vi "Copy Test.vi"(4 "New ID":string, 6 "Move?":bool, 7 "New Parent ID":string, 8 "error in (no error)":errorcluster, 9 "Insertion Index":i32=-1, 10 "Test ID":string, 11 "Test Executive in":refnum<class "Test Executive.lvclass">) -> (0 "error out":errorcluster, 2 "Test ID out":string, 3 "Test Executive out":refnum<class "Test Executive.lvclass">)   [LabVIEW 2019, in "Test Executive.lvlib" / "Test Executive.lvclass"]
uses:
  <vilib>/gpm_packages/@cs/test-executive/Source/Test Executive/TestExecutive/Test Executive.lvclass
  <vilib>/gpm_packages/@cs/test-executive/Source/Test Executive/Executioner/Executioner.lvclass
  <vilib>/gpm_packages/@cs/test-executive/Source/Test Executive/TestExecutive/Test Executive.lvclass/Test Executive.ctl
  a368e383-e4da-4751-aab3-72c07474878c.vi
  fd6f22e2-1d92-4eb3-b93e-b19a74c7291f.vi
  b72c362c-b0aa-47de-9306-dfc13f43c4ad.vi
  cb6e558c-ce6a-4807-984b-722166e3a381.vi
  3584d46b-2973-4467-aaf0-07419839f110.vi
  <vilib>/gpm_packages/@cs/linked-list/Source/Linked List/ILinkedList/ILinked List.lvclass
  <vilib>/gpm_packages/@cs/linked-list/Source/Linked List/Linked List Ref/Linked List Ref.lvclass
panel:
  out "Data IDs out":variant
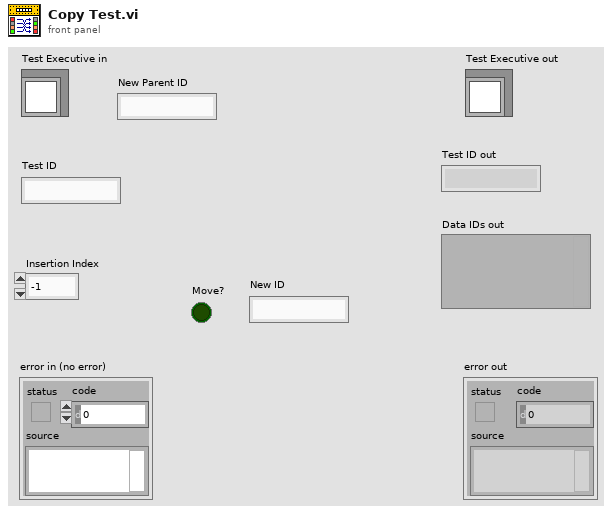
[diagram p1: front panel]
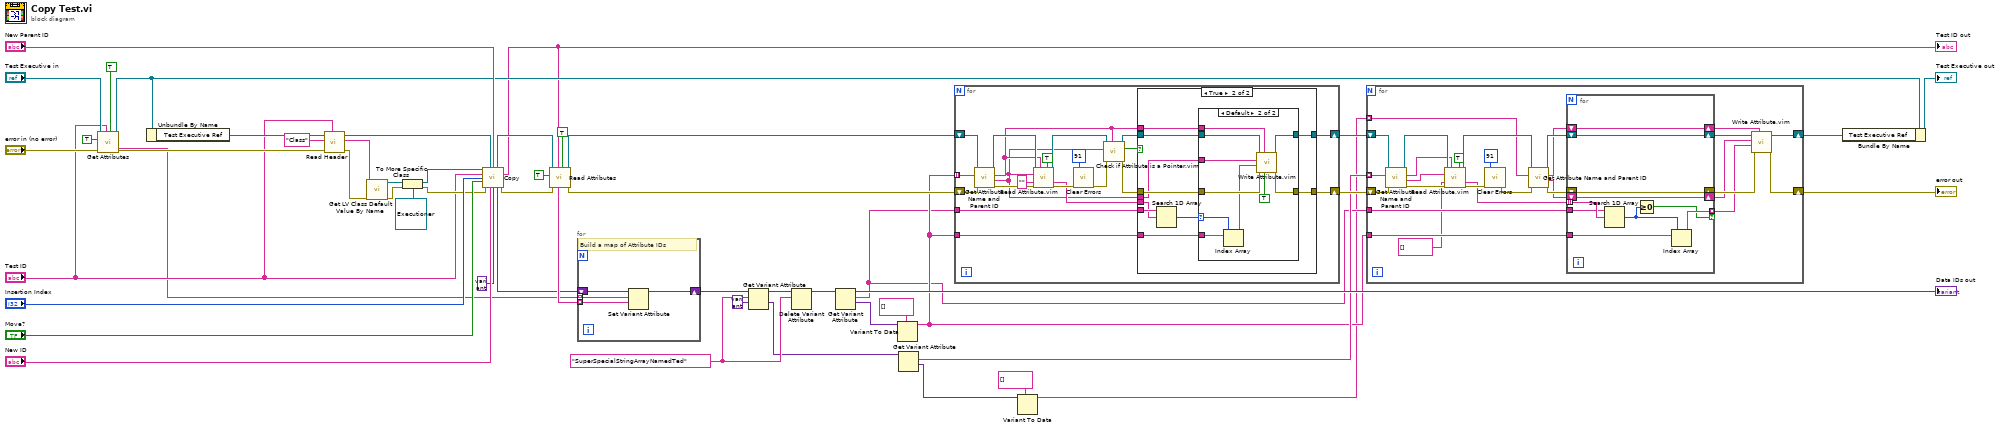
[diagram p0: block diagram]
diagram:
  w12 = "SuperSpecialStringArrayNamedTed" ("name")
  n1 = call-dynamic "Get Attributes.vi"("Flatten Pointer?"=TRUE, "Test ID"="Test ID", "error in (no error)"="error in (no error)", "Include Private?"=TRUE, "Test Executive in"="Test Executive in") -> ("error out"=w34:errorcluster, "Test Executive out"=w36:refnum<class "Test Executive.lvclass">, "Data IDs"=w24:string[])  [unwired: 1 in, 3 out]
  n2 = Unbundle By Name(w36) -> ("Test Executive Ref"=w52:refnum<data-value>)
  n3 = call <vilib>:"Read Header.vi"("Linked List ID"="Test ID", "error in (no error)"=w34, "Header Name"="Class", "Linked List Ref"=w52) -> ("error out"=w40:errorcluster, "Header Value"=w45:string, "Linked List Ref out"=w41:refnum<data-value>)  [unwired: 4 in, 1 out]
  n4 = call <vilib>:"Get LV Class Default Value By Name.vi"("error in (no error)"=w40, "class name"=w45) -> ("error out"=w39:errorcluster, "object"=w44:refnum<class>)  [unwired: 8 in]
  n5 = To More Specific Class(target class=refnum<class "Executioner.lvclass"> refnum ("Test Executive.lvlib:Executioner.lvclass"), reference=w44, error in=w39) -> (specific class reference=w42:refnum<class "Executioner.lvclass">, error out=w38:errorcluster)
  n6 = call-dynamic "Copy.vi"("Executioner in"=w42, "Linked List Ref"=w41, "New Parent ID"="New Parent ID", "Test ID"="Test ID", "Insertion Index"="Insertion Index", "Move?"="Move?", "error in (no error)"=w38, "New ID"="New ID", "Data IDs"=variant) -> ("Linked List Ref out"=w28:refnum<data-value>, "Linked List ID out"=w26:string, "Data IDs out"=w23:variant, "error out"=w27:errorcluster)  [unwired: 3 in]
  "Test ID out" <- w26
  n7 = call <vilib>:"Read Attributes.vi"("Flatten Pointer?"=TRUE, "Linked List ID"=w26, "error in (no error)"=w27, "Include Private?"=TRUE, "Linked List Ref"=w28) -> ("error out"=w19:errorcluster, "Linked List Ref out"=w20:refnum<data-value>, "Data IDs"=w25:string[])  [unwired: 1 in, 3 out]
  n8 = for {
    tunnel: w24 -> [w55] mode=indexing
    tunnel: w25 -> [w54] mode=indexing
    shift-right: [w53] -> w16
    shift-left: w23 -> [w56]
    # "Build a map of Attribute IDs"
    n9 = Set Variant Attribute(Variant=w56, name=w55, value=w54) -> (Variant out=w53:variant)  [unwired: 1 in, 2 out]
  }
  n10 = Get Variant Attribute(Variant=w16, name=w12, default value (empty Variant)=variant ("default value (empty variant)")) -> (duplicate Variant=w15:variant, value=w7:variant)  [unwired: 1 in, 2 out]
  n11 = Delete Variant Attribute(6:w12, 7:w15) -> (3:w14:variant)  [unwired: 1 in, 2 out]
  n12 = Get Variant Attribute(Variant=w14) -> (duplicate Variant=→"Data IDs out":variant, names=w4:string[], values=w18:variant[])  [unwired: 3 in, 1 out]
  n13 = Variant To Data(type=string[] [], Variant=w18) -> (data=w5:string[])  [unwired: 1 in, 1 out]
  n14 = Get Variant Attribute(Variant=w7) -> (names=w6:string[], values=w2:variant[])  [unwired: 3 in, 2 out]
  n15 = for {
    shift-right: [w65] -> w11
    shift-left: w20 -> [w77]
    shift-right: [w63] -> w9
    shift-left: w19 -> [w76]
    tunnel: w4 -> [w60]
    tunnel: w5 -> [w67] mode=indexing
    tunnel: w5 -> [w59]
    n16 = call <vilib>:"Get Attribute Name and Parent ID.vi"("error in (no error)"=w76, "Tag"=w67, "Linked List Ref"=w77) -> ("error out"=w74:errorcluster, "Attribute Name"=w57:string, "Linked List ID"=w58:string, "Linked List Ref out"=w75:refnum<data-value>)  [unwired: 5 in]
    n17 = call "Read Attribute.vim"("Linked List Ref"=w75, "Linked List ID"=w58, "Flatten Pointer?"=TRUE, "Attribute Name"=w57, "Type"="", "error in (no error)"=w74) -> ("Linked List Ref out"=w73:refnum<data-value>, "Attribute"=w62:string, "error out"=w70:errorcluster)  [unwired: 4 in, 3 out]
    n18 = call <vilib>:"Clear Errors.vi"("error in (no error)"=w70, "specific error code to clear (0: all)"=91) -> ("error out"=w69:errorcluster)  [unwired: 4 in, 1 out]
    n19 = call "Check if Attribute is a Pointer.vim"("Linked List ID"=w58, "error in (no error)"=w69, "Attribute Name"=w57, "Linked List Ref"=w73) -> ("error out"=w64:errorcluster, "Pointer?"=w61:bool, "Linked List Ref out"=w66:refnum<data-value>)  [unwired: 3 in, 2 out]
    n20 = case shown="True" w61 {
      tunnel: [w79 w84] -> w65
      tunnel: w66 -> [w79 w85]
      tunnel: [w78 w82] -> w63
      tunnel: w64 -> [w78 w83]
      tunnel: w62 -> [_ w88]
      tunnel: w60 -> [_ w89]
      tunnel: w59 -> [_ w87]
      tunnel: w58 -> [_ w81]
      tunnel: w57 -> [_ w80]
      frame False {
      }
      frame True {
        n21 = Search 1D Array(1D array=w89, element=w88) -> (index of element=w86:i32)  [unwired: 1 in]
        n22 = case shown="Default" w86 {
          selector: w86 -> [_ w100]
          tunnel: w87 -> [_ w101]
          tunnel: w85 -> [w91 w99]
          tunnel: [w91 w98] -> w84
          tunnel: w83 -> [w90 w97]
          tunnel: [w90 w96] -> w82
          tunnel: w81 -> [_ w95]
          tunnel: w80 -> [_ w94]
          frame -1 {
          }
          frame Default {
            n23 = Index Array(array=w101, index=w100) -> (element=w93:string)
            n24 = call "Write Attribute.vim"("Pointer?"=TRUE, "Linked List ID"=w95, "error in (no error)"=w97, "Attribute"=w93, "Attribute Name"=w94, "Linked List Ref"=w99) -> ("error out"=w96:errorcluster, "Linked List Ref out"=w98:refnum<data-value>)  [unwired: 2 in, 2 out]
          }
        }
      }
    }
  }
  n25 = Variant To Data(type=string[] [], Variant=w2) -> (data=w1:string[])  [unwired: 1 in, 1 out]
  n26 = for {
    shift-right: [w116] -> w10
    shift-left: w11 -> [w129]
    shift-right: [w113] -> w8
    shift-left: w9 -> [w128]
    tunnel: w4 -> [w120]
    tunnel: w6 -> [w122] mode=indexing
    tunnel: w5 -> [w119]
    tunnel: w1 -> [w106] mode=indexing
    n27 = call <vilib>:"Get Attribute Name and Parent ID.vi"("error in (no error)"=w128, "Tag"=w122, "Linked List Ref"=w129) -> ("error out"=w126:errorcluster, "Attribute Name"=w103:string, "Linked List ID"=w105:string, "Linked List Ref out"=w127:refnum<data-value>)  [unwired: 5 in]
    n28 = call "Read Attribute.vim"("Linked List Ref"=w127, "Linked List ID"=w105, "Flatten Pointer?"=TRUE, "Attribute Name"=w103, "Type"=string[] [], "error in (no error)"=w126) -> ("Linked List Ref out"=w110:refnum<data-value>, "Attribute"=w121:string[], "error out"=w124:errorcluster)  [unwired: 4 in, 3 out]
    n29 = call <vilib>:"Clear Errors.vi"("error in (no error)"=w124, "specific error code to clear (0: all)"=91) -> ("error out"=w108:errorcluster)  [unwired: 4 in, 1 out]
    n30 = call <vilib>:"Get Attribute Name and Parent ID.vi"("error in (no error)"=w108, "Tag"=w106, "Linked List Ref"=w110) -> ("error out"=w107:errorcluster, "Attribute Name"=w102:string, "Linked List ID"=w104:string, "Linked List Ref out"=w109:refnum<data-value>)  [unwired: 5 in]
    n31 = for {
      tunnel: w121 -> [w139] mode=indexing
      tunnel: w120 -> [w138]
      tunnel: w119 -> [w137]
      shift-right: [w133] -> w117
      shift-left: w109 -> [w133]
      shift-right: [w132] -> w114
      shift-left: w107 -> [w132]
      tunnel: [w135] -> w111 mode=indexing if=w130
      shift-right: [w134] -> w115
      shift-left: w104 -> [w134]
      shift-right: [w131] -> w112
      shift-left: w102 -> [w131]
      n32 = Search 1D Array(1D array=w138, element=w139) -> (index of element=w136:i32)  [unwired: 1 in]
      n33 = Greater Or Equal To 0?(x=w136) -> (x >= 0?=w130:bool)
      n34 = Index Array(array=w137, index=w136) -> (element=w135:string)
    }
    n35 = call "Write Attribute.vim"("Linked List ID"=w115, "error in (no error)"=w114, "Attribute"=w111, "Attribute Name"=w112, "Linked List Ref"=w117) -> ("error out"=w113:errorcluster, "Linked List Ref out"=w116:refnum<data-value>)  [unwired: 3 in, 2 out]
  }
  "error out" <- w8
  n36 = Bundle By Name(cluster=w36, "Test Executive Ref"=w10) -> (→"Test Executive out":refnum<class "Test Executive.lvclass">)
